vi "Subtract.vi"(1 "B":T1={"Array Num"=[1, 2, 3], "Decimal Index"=0, "stop"=FALSE}, 2 "A":T1={"Array Num"=[1, 2, 3], "Decimal Index"=0, "stop"=FALSE}) -> (0 "A-B":T1={"Array Num"=[1, 2, 3], "Decimal Index"=0, "stop"=FALSE})   [LabVIEW 2025]
uses:
  Number.ctl
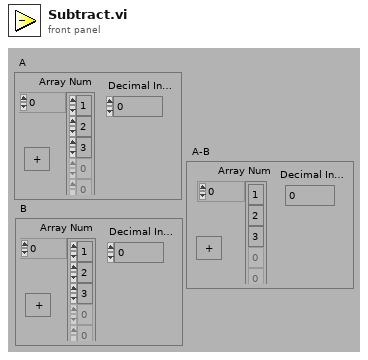
[diagram p1: front panel]
types:
  T1 = typedef "Number.ctl" = cluster{"Array Num":i8[], "Decimal Index":i32, "stop":bool}
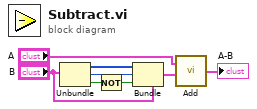
[diagram p0: block diagram]
diagram:
  n1 = Unbundle("B") -> ("Array Num"=w6:i8[], "Decimal Index"=w5:i32, "stop"=w2:bool)
  n2 = Not(x=w2) -> (.not. x?=w3:bool)
  n3 = Bundle(cluster="B", "Array Num"=w6, "Decimal Index"=w5, "stop"=w3) -> (w4:T1)
  n4 = call "Add.vi"("B"=w4, "A"="A") -> ("A+B"=→"A-B":T1)
